vi "Build Constructor.vi"(6 "Project Path":path, 8 "error in (no error)":errorcluster, 9 "Build Specification":string, 10 "Target Name":string, 11 "Builder in":refnum<class "Builder.lvclass">) -> (0 "error out":errorcluster, 3 "Builder out":refnum<class "Builder.lvclass">)   [LabVIEW 2021, in "App-Builder Library.lvlib" / "Builder.lvclass"]
uses:
  Builder.lvclass
  Builder.lvclass/Builder.ctl
  Build specification.ctl
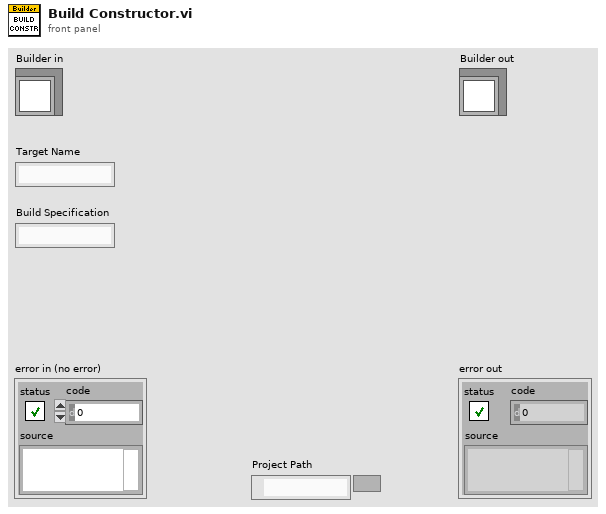
[diagram p1: front panel]
types:
  T1 = typedef "Build specification.ctl" = cluster{"target name":string, "Build specification":string, "Project Path":path}
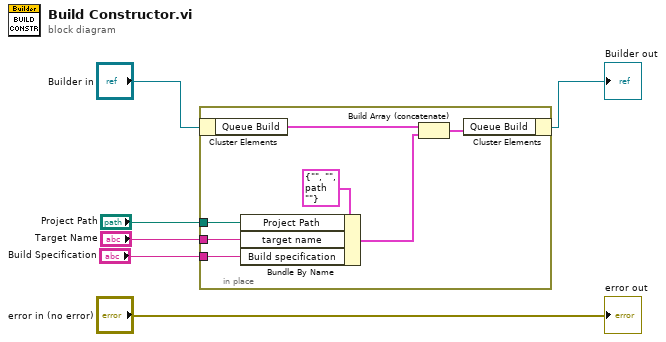
[diagram p0: block diagram]
diagram:
  n1 = in-place {
    in-place-border: "Project Path" -> [w13]
    in-place-border: "Target Name" -> [w12]
    in-place-border: "Build Specification" -> [w11]
    n2 = in-place-cluster #1("Builder in") -> ("Queue Build"=w10:T1[])
    n3 = Bundle By Name(cluster=T1 {"target name"="", "Build specification"="", "Project Path"=path ""} ("Queue Build"), "Project Path"=w13, "target name"=w12, "Build specification"=w11) -> (w7:T1)
    n4 = Build Array (concatenate)(w10, w7) -> (w9:T1[])
    n5 = in-place-cluster #1("Queue Build"=w9) -> (→"Builder out":refnum<class "Builder.lvclass">)
  }
  "error out" <- "error in (no error)"
